vi "Change_Device_Status.vi"(7 "New Status in":bool, 8 "Status/Errors in":refnum<vi>, 9 "Control Parameters [] in":T1[](array[typedef]) {"Aux Byte Value" format="%02x"; "Max Real Value" format="%#_6e"; "Min Real Value" format="%#_6e"; "dReal/dByte" format="%#_6e"; "Byte Value" format="%02x"; "Identifier" format="%02x"}, 10 "Timer parameters in":refnum<vi>, 11 "Device in":refnum<vi>) -> (0 "Status/Errors out":refnum<vi>, 1 "Control Parameters [] out":T1[](array[typedef]) {"Aux Byte Value" format="%02x"; "Max Real Value" format="%#_6e"; "Min Real Value" format="%#_6e"; "dReal/dByte" format="%#_6e"; "Byte Value" format="%02x"; "Identifier" format="%02x"}, 2 "Timer parameters out":refnum<vi>, 3 "Device out":refnum<vi>, 5 "New Status out":bool)   [LabVIEW 2010]
uses:
  Controls/Control_Parameters.ctl
  Controls/Master.ctl
  Controls/Device_Elements.ctl
  Controls/Get_Set_Device_Options.ctl
  Controls/Status_Errors_Elements.ctl
  Controls/Get_Set_Timer_Options.ctl
  Controls/Timer_Elements.ctl
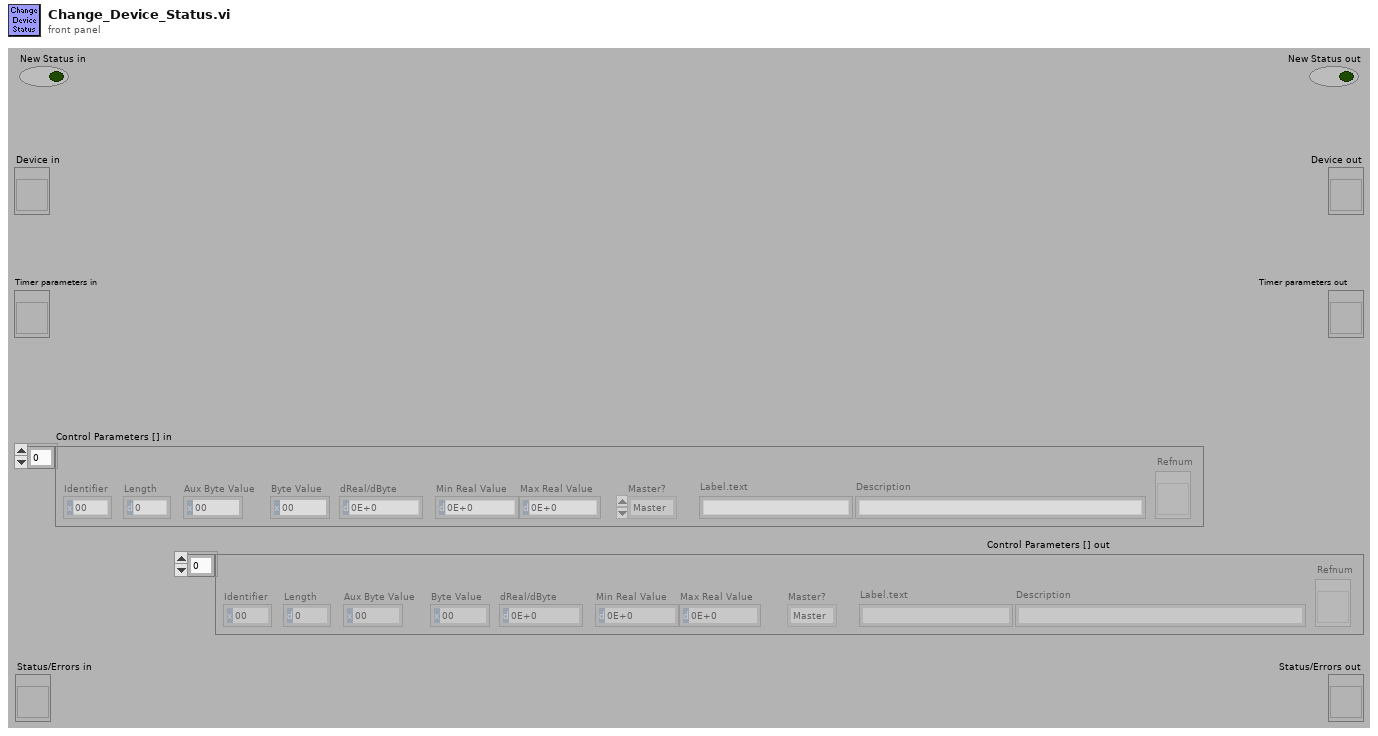
[diagram p1: front panel]
types:
  T1 = typedef "Control_Parameters.ctl" = cluster{"Identifier":u8, "Length":u16, "Byte Value":u32, "dReal/dByte":dbl, "Min Real Value":dbl, "Max Real Value":dbl, "Master?":T2, "Label.text":string, "Description":string, "Refnum":refnum<vi>, "Aux Byte Value":u32}
  T2 = typedef "Master.ctl" = enum16{"Master", "Slave", "General"}
  T3 = typedef "Get_Set_Device_Options.ctl" = enum16{"Get", "Get cluster", "Set"}
  T4 = typedef "Device_Elements.ctl" = enum16{"Default", "Master?", "Connected?", "Status", "Disconnect?", "Handle", "Version number"}
  T5 = typedef "Device.ctl" = cluster{"Master?":T2, "Connected?":bool, "Status":bool, "Disconnect?":bool, "Handle":u32, "Version number":u32}
  T6 = typedef "Get_Set_Timer_Options.ctl" = enum16{"Get", "Get cluster", "Set", "Set to current time"}
  T7 = typedef "Timer_Elements.ctl" = enum16{"Default", "Current time", "Time screen updated", "Time controls locked", "Time last device check", "Time last data MAS", "Time last data SLV", "Time bad status MAS", "Time bad status SLV", "Time clock error updated", "Time delay screen update", "Time delay controls", "Time delay device check", "Time until MAS status bad", "Time until SLV status bad", "Time until MAS connection bad", "Time until SLV connection bad", "Time delay clock error update"}
  T8 = typedef "Status_Errors_Elements.ctl" = enum16{"Default", "Errors", "Master status", "Slave status", "Master connected?", "Slave connected?", "Master GPS on board?", "Slave GPS on board?", "Master: slave detected?", "Slave: slave detected?", "Last message from master", "Last message from slave", "Master temperature"}
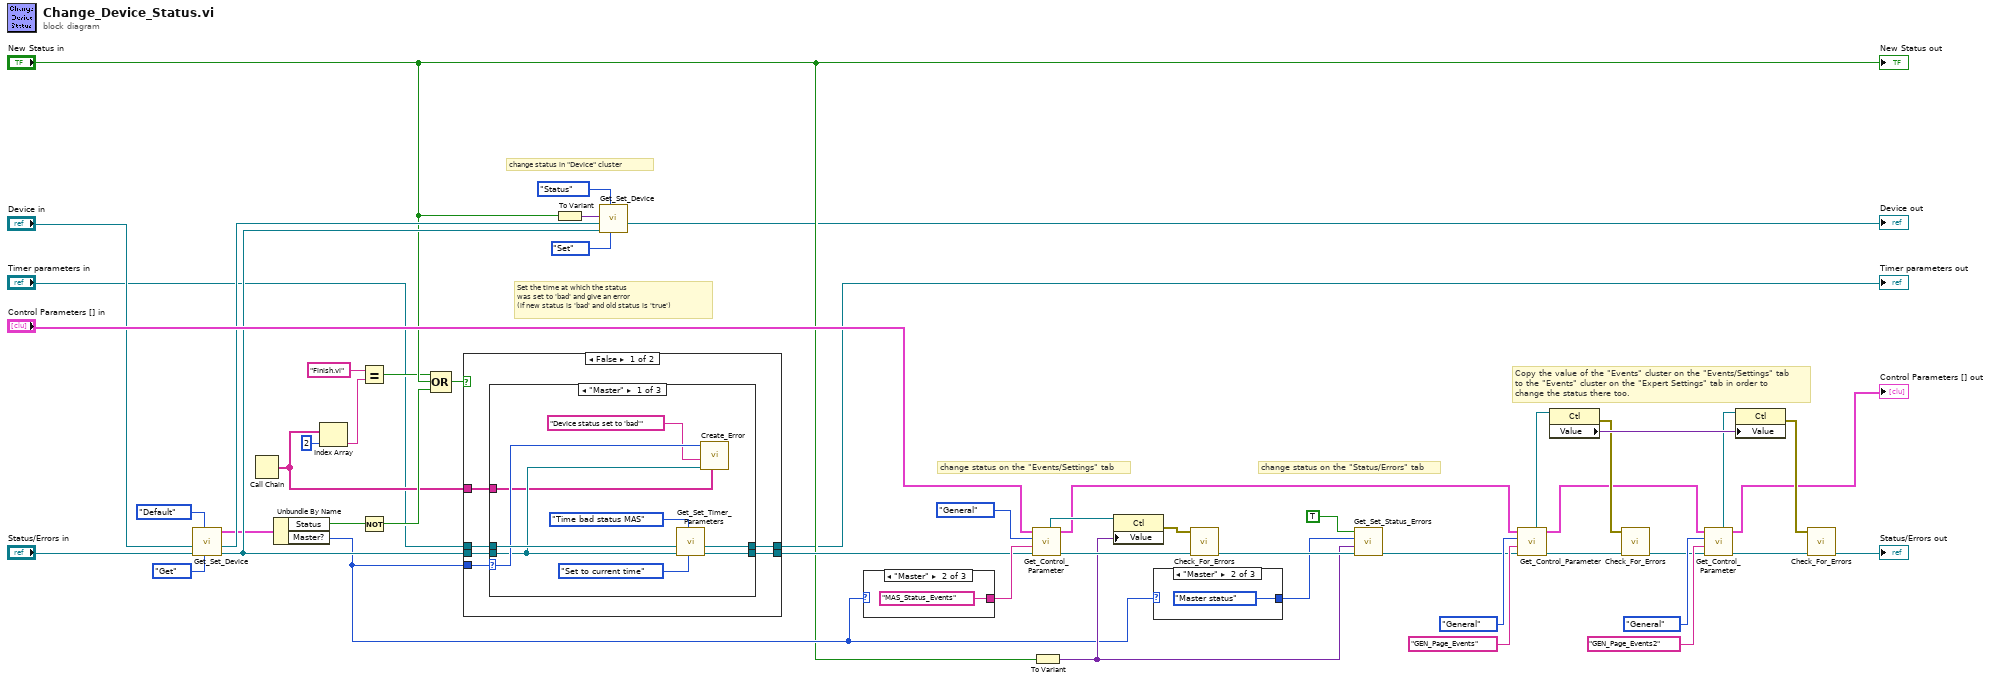
[diagram p0: block diagram]
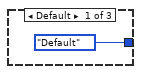
[diagram p2: hidden frame]
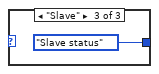
[diagram p3: hidden frame]
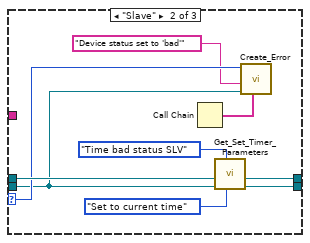
[diagram p4: hidden frame]
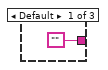
[diagram p7: hidden frame]
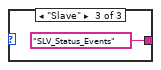
[diagram p8: hidden frame]
diagram:
  # "Set the time at which the status\nwas set to 'bad' and give an error\n(if new status is 'bad' and old status is 'true')"
  # "change status on the \"Status/Errors\" tab"
  # "change status on the \"Events/Settings\" tab"
  # "Copy the value of the \"Events\" cluster on the \"Events/Settings\" tab\nto the \"Events\" cluster on the \"Expert Settings\" tab in order to\nchange the status there too."
  # "change status in \"Device\" cluster"
  n1 = call "Get_Set_Device.vi"("Get/Set"=Get_Set_Device_Options."Get", "Element"=Device_Elements."Default", "Status/Errors in"="Status/Errors in", "Device in"="Device in") -> ("Status/Errors out"=w17:refnum<vi>, "Device out"=w16:refnum<vi>, "Device"=w15:T5)  [unwired: 1 in, 4 out]
  n2 = Call Chain() -> (call chain=w7:string[])
  n3 = Unbundle By Name(w15) -> ("Status"=w12:bool, "Master?"=w14:T2)
  n4 = Index Array(array=w7, index=2) -> (element=w5:string)
  n5 = Equal?(x="Finish.vi", y=w5) -> (x = y?=w3:bool)
  n6 = Not(x=w12) -> (.not. x?=w11:bool)
  n7 = Compound Arithmetic op=OR(w3, "New Status in", w11) -> (w13:bool)
  n8 = case shown="False" w13 {
    tunnel: "Timer parameters in" -> [w56 w79]
    tunnel: [w57 w79] -> w1
    tunnel: w17 -> [w55 w78]
    tunnel: [w54 w78] -> w25
    tunnel: w14 -> [w53 _]
    tunnel: w7 -> [w52 _]
    frame False {
      n9 = case shown="\"Master\"" w53 {
        selector: w53 -> [w63 w72 _]
        tunnel: w56 -> [w66 w75 w77]
        tunnel: [w65 w74 w77] -> w57
        tunnel: w55 -> [w62 w71 w76]
        tunnel: [w64 w73 w76] -> w54
        tunnel: w52 -> [w58 _ _]
        frame "Master" {
          n10 = call "Get_Set_Timer_Parameters.vi"("Get/Set"=Get_Set_Timer_Options."Set to current time", "Element"=Timer_Elements."Time bad status MAS", "Status/Errors in"=w62, "Timer parameters in"=w66) -> ("Status/Errors out"=w64:refnum<vi>, "Timer parameters out"=w65:refnum<vi>)  [unwired: 2 in, 4 out]
          n11 = call "Create_Error.vi"("Call chain"=w58, "Status/Errors in"=w62, "HiSPARC error"="Device status set to 'bad'", "Master?"=w63) -> ()  [unwired: 2 in, 6 out]
        }
        frame "Slave" {
          n12 = Call Chain() -> (call chain=w70:string[])
          n13 = call "Get_Set_Timer_Parameters.vi"("Get/Set"=Get_Set_Timer_Options."Set to current time", "Element"=Timer_Elements."Time bad status SLV", "Status/Errors in"=w71, "Timer parameters in"=w75) -> ("Status/Errors out"=w73:refnum<vi>, "Timer parameters out"=w74:refnum<vi>)  [unwired: 2 in, 4 out]
          n14 = call "Create_Error.vi"("Call chain"=w70, "Status/Errors in"=w71, "HiSPARC error"="Device status set to 'bad'", "Master?"=w72) -> ()  [unwired: 2 in, 6 out]
        }
        frame Default {
        }
      }
    }
    frame True {
    }
  }
  "Timer parameters out" <- w1
  n15 = To Variant(anything="New Status in") -> (Variant=w20:variant)
  n16 = call "Get_Set_Device.vi"("Get/Set"=Get_Set_Device_Options."Set", "Element"=Device_Elements."Status", "Status/Errors in"=w17, "Device in"=w16, "Value in"=w20) -> ("Device out"=→"Device out":refnum<vi>)  [unwired: 6 out]
  n17 = case shown="\"Master\"" w14 {
    tunnel: ["" "MAS_Status_Events" ("Label.text in") "SLV_Status_Events" ("Label.text in")] -> w41
    frame Default {
    }
    frame "Master" {
    }
    frame "Slave" {
    }
  }
  n18 = call "Get_Control_Parameter.vi"("Status/Errors in"=w25, "Label.text in"=w41, "Master?"=Master."General", "Control Parameters [] in"="Control Parameters [] in") -> ("Status/Errors out"=w35:refnum<vi>, "Control Parameters [] out"=w31:T1[], "Refnum"=w42:refnum<vi>)  [unwired: 5 out]
  n19 = To Variant(anything="New Status in") -> (Variant=w28:variant)
  n20 = property class="Ctl"(reference=w42, "Value"=w28) -> (error out=w34:errorcluster)  [unwired: 1 in, 1 out]
  n21 = case shown="\"Master\"" w14 {
    tunnel: [Status_Errors_Elements."Default" ("Element") Status_Errors_Elements."Master status" ("Element") Status_Errors_Elements."Slave status" ("Element")] -> w27
    frame Default {
    }
    frame "Master" {
    }
    frame "Slave" {
    }
  }
  n22 = call "Check_For_Errors.vi"("Status/Errors in"=w35, "error in"=w34) -> ("Status/Errors out"=w30:refnum<vi>)  [unwired: 9 out]
  n23 = call "Get_Set_Status_Errors.vi"("Status/Errors in"=w30, "Value in"=w28, "Element"=w27, "Set?"=TRUE) -> ("Status/Errors out"=w29:refnum<vi>)  [unwired: 7 out]
  n24 = call "Get_Control_Parameter.vi"("Status/Errors in"=w29, "Label.text in"="GEN_Page_Events", "Master?"=Master."General", "Control Parameters [] in"=w31) -> ("Status/Errors out"=w39:refnum<vi>, "Control Parameters [] out"=w36:T1[], "Refnum"=w50:refnum<vi>)  [unwired: 5 out]
  n25 = property class="Ctl"(reference=w50) -> (error out=w37:errorcluster, "Value"=w49:variant)  [unwired: 1 in, 1 out]
  n26 = call "Check_For_Errors.vi"("Status/Errors in"=w39, "error in"=w37) -> ("Status/Errors out"=w38:refnum<vi>)  [unwired: 9 out]
  n27 = call "Get_Control_Parameter.vi"("Status/Errors in"=w38, "Label.text in"="GEN_Page_Events2", "Master?"=Master."General", "Control Parameters [] in"=w36) -> ("Status/Errors out"=w46:refnum<vi>, "Control Parameters [] out"=→"Control Parameters [] out":T1[], "Refnum"=w44:refnum<vi>)  [unwired: 5 out]
  n28 = property class="Ctl"(reference=w44, "Value"=w49) -> (error out=w45:errorcluster)  [unwired: 1 in, 1 out]
  n29 = call "Check_For_Errors.vi"("Status/Errors in"=w46, "error in"=w45) -> ("Status/Errors out"=→"Status/Errors out":refnum<vi>)  [unwired: 9 out]
  "New Status out" <- "New Status in"
